vi "request change motor state.vi"(9 "messageHandler in":T2 {"params"."controlChannels"."ballControl" items=["Module6/output0", "Module6/output1", "Module6/output2", "Module6/output3", "Not-Used"]; "params"."controlChannels"."butterflyControl" items=["Module6/output0", "Module6/output1", "Module6/output2", "Module6/output3", "Not-Used"]; "params"."controlChannels"."speedControl" items=["Module6/output0", "Module6/output1", "Module6/output2", "Module6/output3", "Not-Used"]}, 10 "new output":bool, 11 "Queues in":T1) -> (3 "messageHandler out":T2 {"params"."controlChannels"."ballControl" items=["Module6/output0", "Module6/output1", "Module6/output2", "Module6/output3", "Not-Used"]; "params"."controlChannels"."butterflyControl" items=["Module6/output0", "Module6/output1", "Module6/output2", "Module6/output3", "Not-Used"]; "params"."controlChannels"."speedControl" items=["Module6/output0", "Module6/output1", "Module6/output2", "Module6/output3", "Not-Used"]})   [LabVIEW 2018]
uses:
  type defs/message handler data.ctl
  customVI/liveData/state.ctl
  type defs/Queues.ctl
  <vilib>/Utility/error.llb/Error Cluster From Error Code.vi
  supporting VIs/polymorphic VIs/enqueue for user interface.vi
  supporting VIs/polymorphic VIs/enqueue for message handler.vi
  <vilib>/ErrorRing/Error Ring.xnode
panel:
  out "Interlocks OK":bool
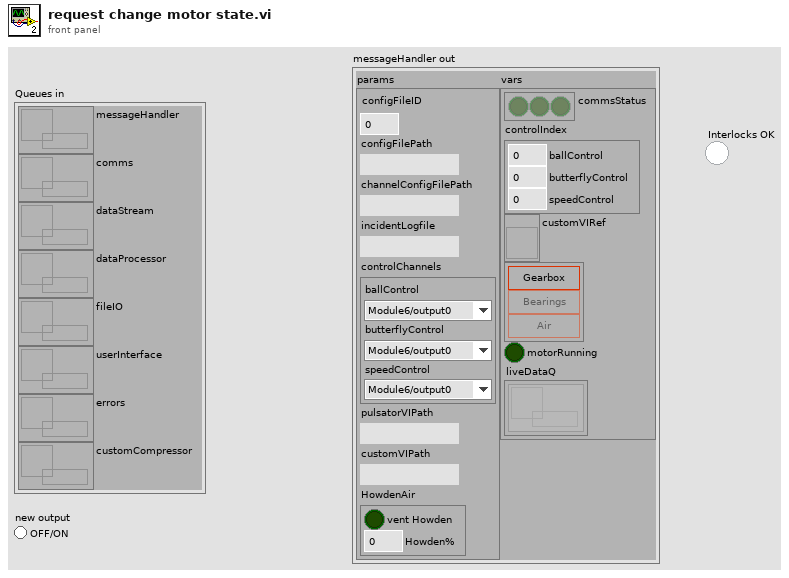
[diagram p1: front panel]
types:
  T1 = typedef "Queues.ctl" = cluster{"messageHandler":refnum<queue>, "comms":refnum<queue>, "dataStream":refnum<queue>, "dataProcessor":refnum<queue>, "fileIO":refnum<queue>, "userInterface":refnum<queue>, "errors":refnum<queue>, "customCompressor":refnum<queue>}
  T2 = typedef "message handler data.ctl" = cluster{"params":cluster{"configFileID":u32, "configFilePath":path, "channelConfigFilePath":path, "incidentLogfile":path, "controlChannels":cluster{"ballControl":u16, "butterflyControl":u16, "speedControl":u16}, "pulsatorVIPath":path, "customVIPath":path, "HowdenAir":cluster{"vent Howden":bool, "Howden%":dbl}}, "vars":cluster{"commsStatus":bool[], "controlIndex":cluster{"ballControl":u16, "butterflyControl":u16, "speedControl":u16}, "customVIRef":refnum<vi>, "Interlocks":cluster{"gearboxOil":bool, "bearingOil":bool, "gearboxAir":bool}, "motorRunning":bool, "liveDataQ":refnum<queue>[]}}
  T3 = cluster{"gearboxOil":bool, "bearingOil":bool, "gearboxAir":bool}
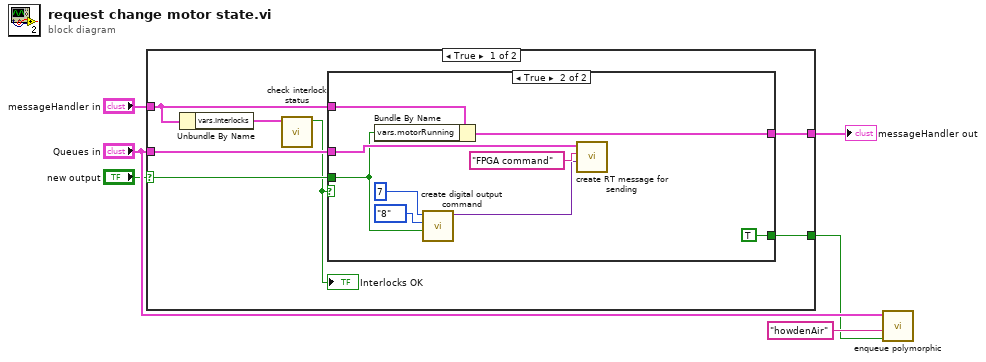
[diagram p0: block diagram]
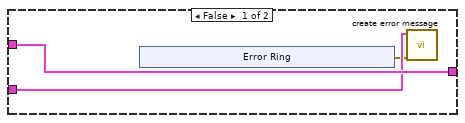
[diagram p2: hidden frame]
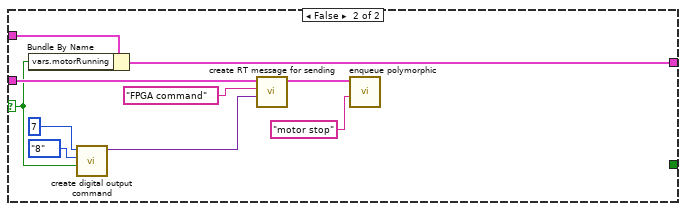
[diagram p3: hidden frame]
diagram:
  n1 = case shown="True" "new output" {
    selector: "new output" -> [w11 w33]
    tunnel: "Queues in" -> [w13 w38]
    tunnel: "messageHandler in" -> [w9 w35]
    tunnel: [w12 w34] -> w6
    tunnel: [w7 _] -> w1
    frame True {
      n2 = Unbundle By Name(w9) -> ("vars.Interlocks"=w8:T3)
      n3 = call "check interlock status.vi"("Interlocks"=w8) -> ("interlocksOK"=w10:bool)  [unwired: 10 in]
      "Interlocks OK" <- w10
      n4 = case shown="True" w10 {
        tunnel: w13 -> [w15 w28]
        tunnel: w9 -> [w16 w25]
        tunnel: [w16 w24] -> w12
        tunnel: w11 -> [_ w23]
        tunnel: [_ TRUE] -> w7
        frame False {
          n5 = xnode "Error Ring"() -> ("error out"=w14:errorcluster)
          n6 = call "create error message.vi"("error in (no error)"=w14, "queues"=w15) -> ()  [unwired: 10 in]
        }
        frame True {
          n7 = Bundle By Name(cluster=w25, "vars.motorRunning"=w23) -> (w24:T2)
          n8 = call "create digital output command.vi"("new output"=w23, "module"=enum16{"7", "8"}."8", "Index"=7) -> ("command message"=w26:variant)  [unwired: 8 in]
          n9 = call "create RT message for sending.vi"("RT data"=w26, "RT message"="FPGA command", "Queues in"=w28) -> ()  [unwired: 8 in, 1 out]
        }
      }
    }
    frame False {
      n10 = Bundle By Name(cluster=w35, "vars.motorRunning"=w33) -> (w34:T2)
      n11 = call "create digital output command.vi"("new output"=w33, "module"=enum16{"7", "8"}."8", "Index"=7) -> ("command message"=w36:variant)  [unwired: 8 in]
      n12 = call "create RT message for sending.vi"("RT data"=w36, "RT message"="FPGA command", "Queues in"=w38) -> ("Queues out"=w32:T1)  [unwired: 8 in]
      n13 = call-poly "enqueue polymorphic.vi"("message"="motor stop", "Queues"=w32) -> ()  [unwired: 9 in, 1 out]
    }
  }
  "messageHandler out" <- w6
  n14 = call-poly "enqueue polymorphic.vi"("data"=w1, "message"="howdenAir", "Queues"="Queues in") -> ()  [unwired: 8 in, 1 out]
